vi "Kafka_SendData.vi"(8 "error in (no error)":errorcluster, 9 "Events":T1[](array[typedef]), 10 "Partition":i32, 11 "Producer Handle":string="localhost:9092") -> (0 "error out":errorcluster, 3 "Producer Handle":string)   [LabVIEW 2019]
uses:
  KafkaConsumerEvent.ctl
  VS2017/KafkaLVLib/x64/Debug/KafkaLVLib.dll
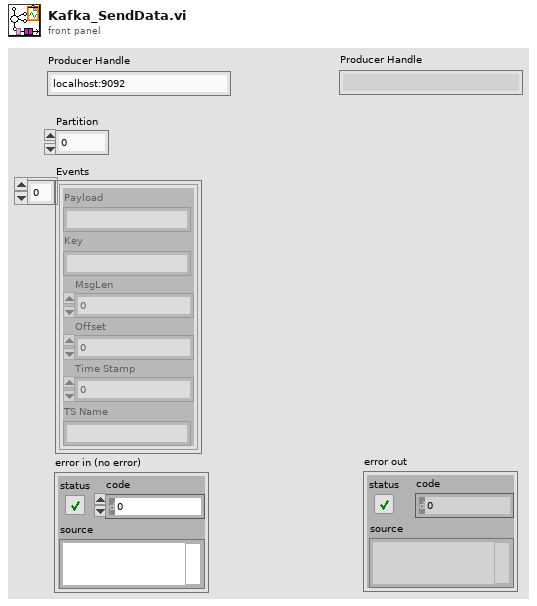
[diagram p1: front panel]
types:
  T1 = typedef "KafkaConsumerEvent.ctl" = cluster{"Payload":string, "Key":string, "MsgLen":u64, "Offset":i64, "Time Stamp":i64, "TS Name":string}
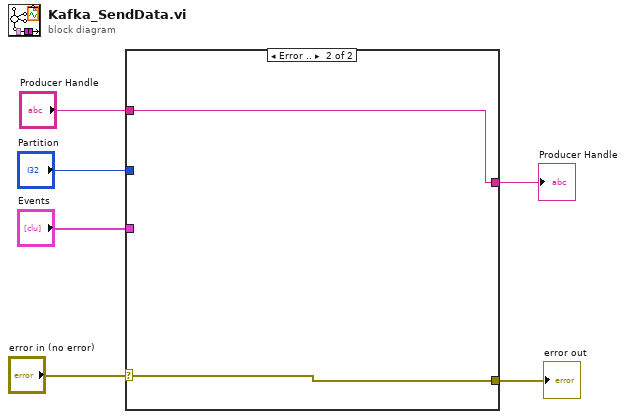
[diagram p0: block diagram]
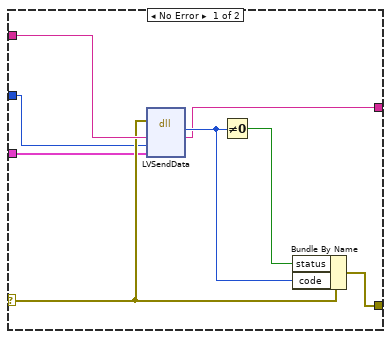
[diagram p2: hidden frame]
diagram:
  n1 = case shown="Error .." "error in (no error)" {
    selector: "error in (no error)" -> [w10 w16]
    tunnel: "Producer Handle" -> [w11 w15]
    tunnel: [w12 w16] -> w4
    tunnel: [w9 w15] -> w3
    tunnel: "Events" -> [w8 _]
    tunnel: "Partition" -> [w7 _]
    frame No Error {
      n2 = dll-call lib="C:/Users/schandho/OneDrive - National Instruments/Research/Virtualization/SemiADV/KafkaLVLib/VS2017/KafkaLVLib/x64/Debug/KafkaLVLib.dll" fn="LVSendData"(error in=w10, "producerhandle"=w11, "partition"=w7, "events"=w8) -> ("error"=w13:i32, "producerhandle"=w9:string)  [unwired: 4 in, 2 out]
      n3 = Not Equal To 0?(x=w13) -> (x != 0?=w14:bool)
      n4 = Bundle By Name(cluster=w10, "status"=w14, "code"=w13) -> (w12:errorcluster)
    }
    frame Error {
    }
  }
  "error out" <- w4
  "Producer Handle" <- w3
